vi "Update Limit.vi"(8 "error in (no error)":errorcluster, 9 "Upper Range":dbl, 10 "Lower Range":dbl, 11 "XYGraphOverview in":refnum<class "XYGraphOverview.lvclass">) -> (0 "error out":errorcluster, 3 "XYGraphOverview out":refnum<class "XYGraphOverview.lvclass">)   [LabVIEW 2020, in "XYGraphOverview.lvlib" / "XYGraphOverview.lvclass"]
uses:
  XYGraphOverview.lvclass
  Caller User Event Data.ctl
  Command.ctl
  X Range Change User Event Data.ctl
  XYGraphOverview.lvclass/XYGraphOverview.ctl
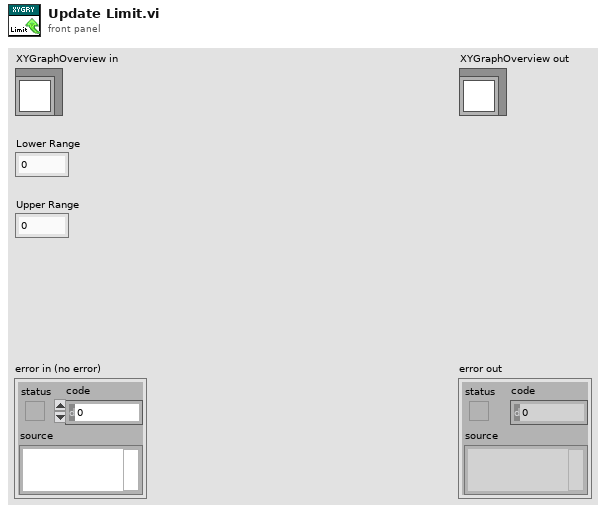
[diagram p1: front panel]
types:
  T1 = typedef "XYGraphOverview.lvlib/XYGraphOverview.lvclass/X Range Change User Event Data.ctl" = cluster{"Lower Range":dbl, "Upper Range":dbl, "All":bool}
  T2 = typedef "XYGraphOverview.lvlib/XYGraphOverview.lvclass/Caller User Event Data.ctl" = cluster{"Command":T3, "Data":variant}
  T3 = typedef "XYGraphOverview.lvlib/XYGraphOverview.lvclass/Command.ctl" = enum16{"Update Data", "Update Limit", "Zoom"}
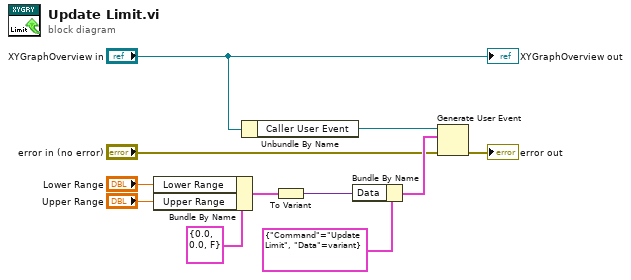
[diagram p0: block diagram]
diagram:
  n1 = Bundle By Name(cluster=T1 {"Lower Range"=0.0, "Upper Range"=0.0, "All"=FALSE} ("X Range Change User Event Data"), "Lower Range"="Lower Range", "Upper Range"="Upper Range") -> (w3:T1)
  n2 = Unbundle By Name("XYGraphOverview in") -> ("Caller User Event"=w11:refnum<user-event>)
  n3 = To Variant(anything=w3) -> (Variant=w9:variant)
  n4 = Bundle By Name(cluster=T2 {"Command"=enum."Update Limit", "Data"=variant} ("event data"), "Data"=w9) -> (w8:T2)
  n5 = Generate User Event(user event=w11, event data cluster=w8, error in="error in (no error)") -> (error out=→"error out":errorcluster)  [unwired: 1 in, 1 out]
  "XYGraphOverview out" <- "XYGraphOverview in"
